vi "Configure NI-SWITCH Custom Device.vi"(8 "error in":errorcluster, 9 "resource":string, 10 "topologies":string[](array[string]), 11 "ni-switch custom device in":T1 format="%.0x") -> (0 "error out":errorcluster, 3 "ni-switch custom device out":T1 format="%.0x")   [LabVIEW 2017, in "NI-SWITCH Scripting.lvlib"]
uses:
  NI-SWITCH Scripting.lvlib
  <vilib>/NI Veristand/Custom Device API/Custom Device Item Ref.ctl
  Properties/NI-SWITCH All Properties.ctl
  <vilib>/NI VeriStand/Custom Device API/Custom Device API.lvlib
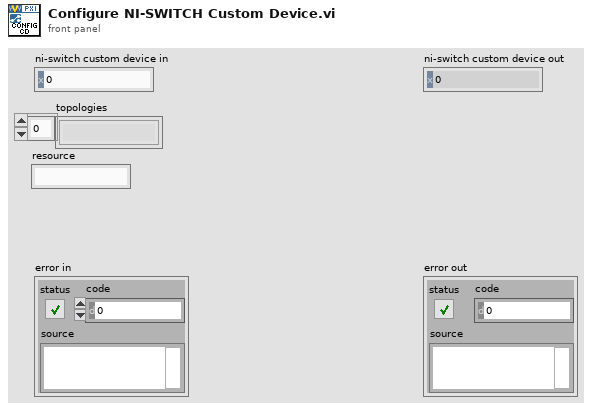
[diagram p1: front panel]
types:
  T1 = typedef "Custom Device API.lvlib/Custom Device Item Ref.ctl" = u64
  T2 = typedef "NI-SWITCH Scripting.lvlib/NI-SWITCH All Properties.ctl" = cluster{"Resource":string, "Topology":string, "Description":string}
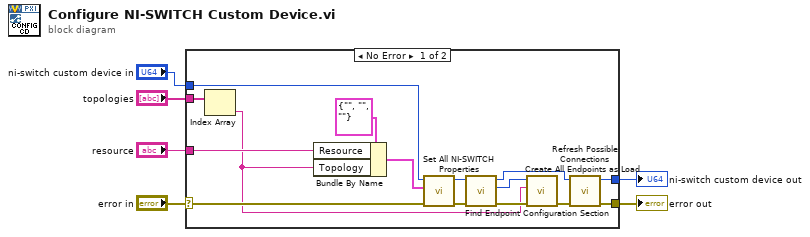
[diagram p0: block diagram]
diagram:
  n1 = case shown="No Error" "error in" {
    selector: "error in" -> [w10 w22]
    tunnel: "resource" -> [w21 _]
    tunnel: [w8 w22] -> w5
    tunnel: [w9 w23] -> w4
    tunnel: "topologies" -> [w12 _]
    tunnel: "ni-switch custom device in" -> [w11 w23]
    frame No Error {
      n2 = Index Array(array=w12) -> (element=w7:string)  [unwired: 1 in]
      n3 = Bundle By Name(cluster=T2 {"Resource"="", "Topology"="", "Description"=""} ("SLSC Switch All Properties"), "Resource"=w21, "Topology"=w7) -> (w13:T2)
      n4 = call "Set All NI-SWITCH Properties.vi"("error in"=w10, "properties"=w13, "ni-switch custom device in"=w11) -> ("error out"=w20:errorcluster, "ni-switch custom device out"=w15:T1)  [unwired: 7 in]
      n5 = call "Find Endpoint Configuration Section.vi"("error in"=w20, "ni-switch custom device in"=w15) -> ("error out"=w19:errorcluster, "endpoint configuration"=w18:T1, "ni-switch custom device out"=w17:T1)  [unwired: 7 in]
      n6 = call "Create All Endpoints as Load.vi"("error in"=w19, "topology"=w7, "endpoint configuration in"=w18) -> ("error out"=w16:errorcluster)  [unwired: 7 in, 1 out]
      n7 = call "Refresh Possible Connections.vi"("error in"=w16, "ni-switch custom device in"=w17) -> ("error out"=w8:errorcluster, "ni-switch custom device out"=w9:T1)  [unwired: 8 in]
    }
    frame Error {
    }
  }
  "error out" <- w5
  "ni-switch custom device out" <- w4
